vi "uTransport_IsValid.vi"(8 "error in (no error)":errorcluster, 11 "uTransport in":refnum<class "uTransport.lvclass">) -> (0 "error out":errorcluster, 2 "IsValid?":bool, 3 "uTransport out":refnum<class "uTransport.lvclass">)   [LabVIEW 2023, in "uLib.lvlib" / "uTransport.lvclass"]
doc: "Returns true if the refnum is still valid."
uses:
  uTransport.lvclass
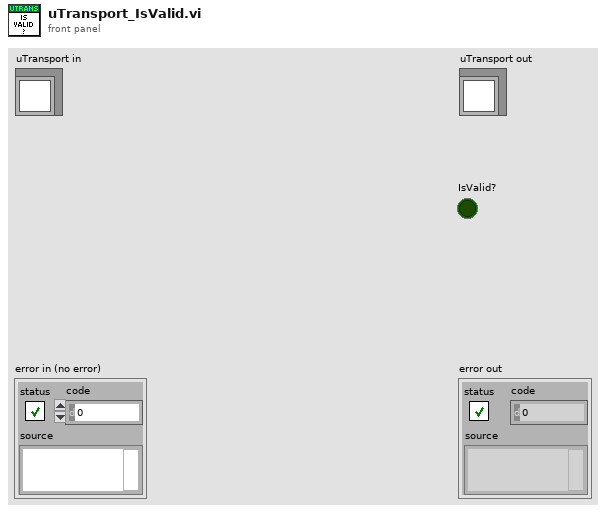
[diagram p1: front panel]
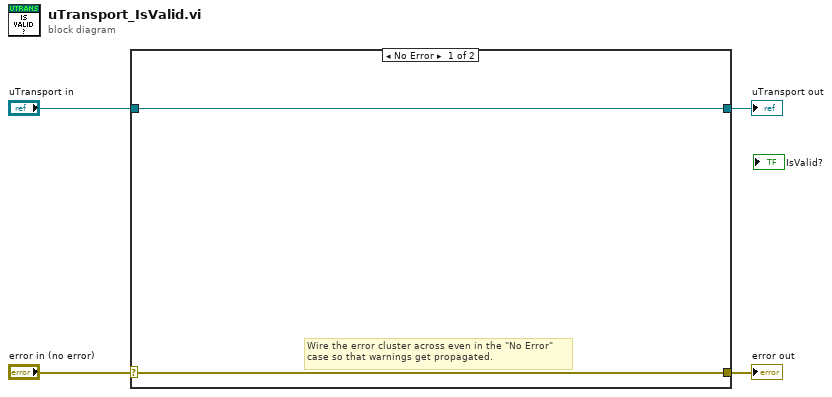
[diagram p0: block diagram]
diagram:
  n1 = case shown="No Error" "error in (no error)" {
    selector: "error in (no error)" -> [w5 w8]
    tunnel: [w5 w8] -> w3
    tunnel: [w6 w7] -> w1
    tunnel: "uTransport in" -> [w6 w7]
    frame No Error {
      # "Wire the error cluster across even in the \"No Error\"\ncase so that warnings get propagated."
    }
    frame Error {
    }
  }
  "error out" <- w3
  "uTransport out" <- w1
